vi "Waveforms.Process.vi"(0 "Data":dbl[](array[numeric]), 1 "Waveform.Ref":T1, 2 "WaveformGraph.Ref":refnum<vi>, 3 "Reset?":bool, 5 "dt":dbl, 7 "offset from start (samples)":u64, 9 "t0 at start":timestamp, 11 "error in (no error)":errorcluster, 12 "Waveforms":T5) -> (15 "error out":errorcluster)   [LabVIEW 2015, in "Station.Execution.lvlib"]
uses:
  Station.Execution.lvlib
  <vilib>/NI Veristand/Execution/WaveformStreaming/WaveformStreamSpecification.ctl
  NationalInstruments.VeriStand.ClientAPI
  <vilib>/NI Veristand/Execution/WaveformStreaming/Registered Waveform Streams Data Event Refnum (DBL).ctl
  <vilib>/NI Veristand/Execution/WaveformStreaming/Waveform Data Watcher Event Data (DBL).ctl
  <vilib>/NI Veristand/Execution/WaveformStreaming/WaveformDataWatcherDBL.ctl
  <vilib>/NI Veristand/Execution/WaveformStreaming/WaveformStreamingAPI.ctl
  <vilib>/NI Veristand/Execution/WaveformStreaming/NI_VS Waveform Streaming Interface.lvlib
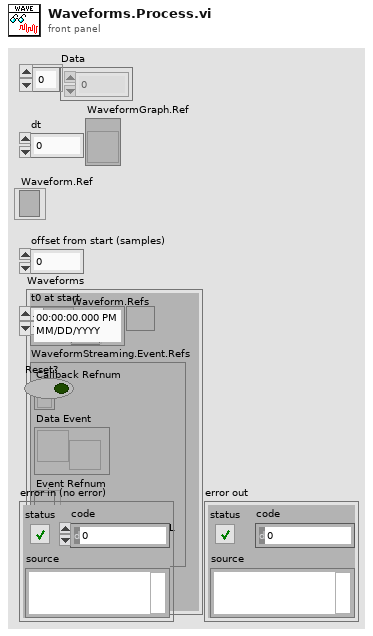
[diagram p1: front panel]
types:
  T1 = typedef "NI_VS Waveform Streaming Interface.lvlib/WaveformStreamSpecification.ctl" = refnum<k24>
  T2 = typedef "NI_VS Waveform Streaming Interface.lvlib/Registered Waveform Streams Data Event Refnum (DBL).ctl" = cluster{"Callback Refnum":refnum<k27>, "Data Event":refnum<user-event>, "Event Refnum":refnum<event-registration>, "WaveformDataWatcherDBL":T3}
  T3 = typedef "NI_VS Waveform Streaming Interface.lvlib/WaveformDataWatcherDBL.ctl" = refnum<k24>
  T4 = typedef "NI_VS Waveform Streaming Interface.lvlib/WaveformStreamingAPI.ctl" = refnum<k24>
  T5 = cluster{"Waveform.Refs":T1[], "WaveformStreaming.Event.Refs":T2, "WaveformStreaming.Ref":T4}
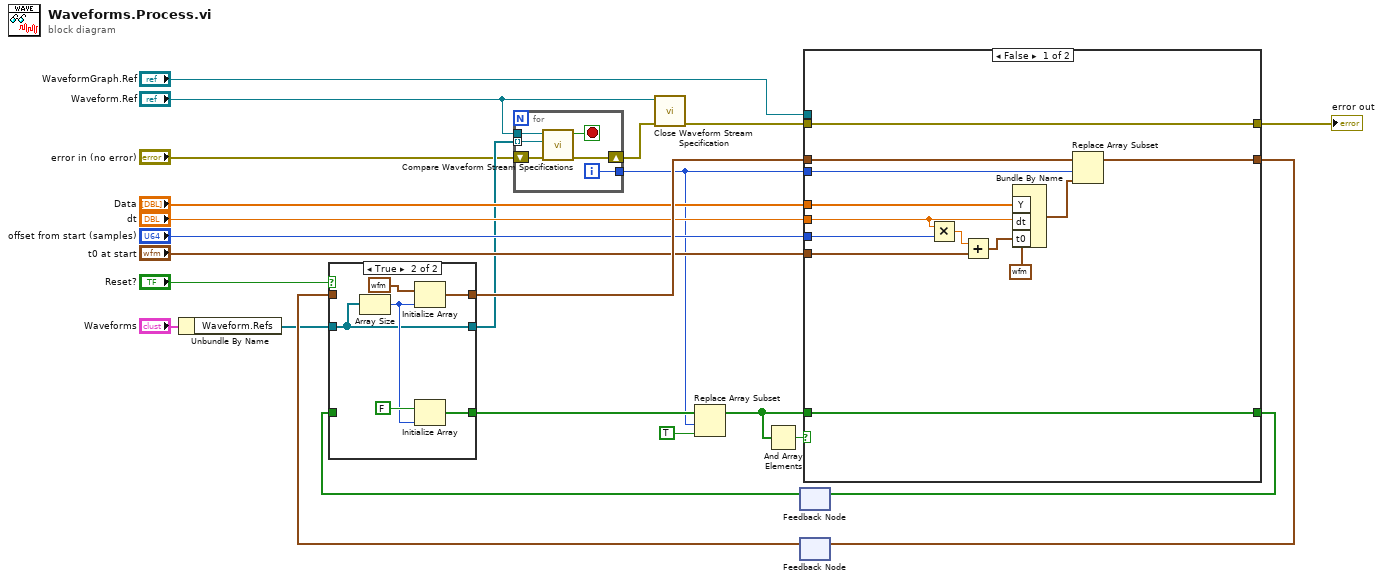
[diagram p0: block diagram]
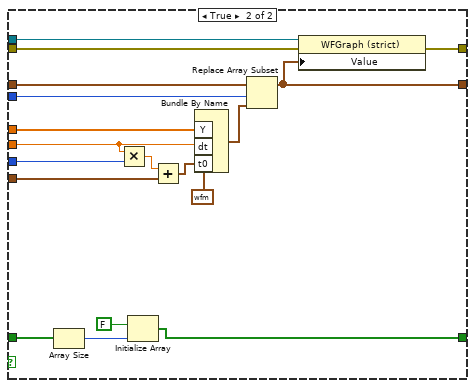
[diagram p3: hidden frame]
diagram:
  n1 = Unbundle By Name("Waveforms") -> ("Waveform.Refs"=w6:T1[])
  n2 = feedback #1() -> (w23:bool[])  [unwired: 1 in]
  n3 = feedback #2() -> (w24:waveform(dbl)[])  [unwired: 1 in]
  n4 = case shown="True" "Reset?" {
    tunnel: w6 -> [w25 w28]
    tunnel: [w27 w31] -> w19
    tunnel: [w26 w30] -> w20
    tunnel: w23 -> [w27 _]
    tunnel: w24 -> [w26 _]
    tunnel: [w25 w28] -> w5
    frame False {
    }
    frame True {
      n5 = Array Size(array=w28) -> (size(s)=w29:i32)
      n6 = Initialize Array(waveform(dbl) {"t0"=timestamp(0 s since 1904-01-01), "dt"=1.0, "Y"=[]} ("waveform"), w29) -> (w30:waveform(dbl)[])
      n7 = Initialize Array(FALSE, w29) -> (w31:bool[])
    }
  }
  n8 = for {
    tunnel: w5 -> [w39] mode=indexing
    tunnel: [w37] -> w4
    tunnel: "Waveform.Ref" -> [w36]
    shift-right: [w34] -> w1
    shift-left: "error in (no error)" -> [w35]
    i -> [w37]
    stop <- w38 stop-if-true
    n9 = call <vilib>:"Compare Waveform Stream Specifications.vi"("error in (no error)"=w35, "WaveformStreamSpecification to compare"=w39, "WaveformStreamSpecification"=w36) -> ("error out"=w34:errorcluster, "equivalent?"=w38:bool)  [unwired: 7 in]
  }
  n10 = call <vilib>:"Close Waveform Stream Specification.vi"("error in (no error)"=w1, "WaveformStreamSpecification"="Waveform.Ref") -> ("error out"=w10:errorcluster)  [unwired: 9 in]
  n11 = Replace Array Subset(array=w19, new element=TRUE ("new element/subarray"), index=w4) -> (w13:bool[])
  n12 = And Array Elements(Boolean array=w13) -> (logical AND=w12:bool)
  n13 = case shown="False" w12 {
    tunnel: w13 -> [w52 w63]
    tunnel: [w52 w60] -> w22
    tunnel: w4 -> [w51 w68]
    tunnel: w20 -> [w50 w70]
    tunnel: [w49 w69] -> w21
    tunnel: "Data" -> [w48 w67]
    tunnel: "dt" -> [w47 w66]
    tunnel: "t0 at start" -> [w46 w64]
    tunnel: "offset from start (samples)" -> [w45 w65]
    tunnel: w10 -> [w44 w59]
    tunnel: [w44 w58] -> w9
    tunnel: "WaveformGraph.Ref" -> [_ w57]
    frame False {
      n14 = Multiply(x=w47, y=w45) -> (x*y=w42:dbl)
      n15 = Add(x=w42, y=w46) -> (x+y=w43:timestamp)
      n16 = Bundle By Name(cluster=waveform(dbl) {"t0"=timestamp(0 s since 1904-01-01), "dt"=1.0, "Y"=[]} ("waveform"), "Y"=w48, "dt"=w47, "t0"=w43) -> (w40:waveform(dbl))
      n17 = Replace Array Subset(array=w50, new element=w40, index=w51) -> (w49:waveform(dbl)[])
    }
    frame True {
      n18 = Array Size(array=w63) -> (size(s)=w61:i32)
      n19 = Multiply(x=w66, y=w65) -> (x*y=w55:dbl)
      n20 = Initialize Array(FALSE, w61) -> (w60:bool[])
      n21 = Add(x=w55, y=w64) -> (x+y=w56:timestamp)
      n22 = Bundle By Name(cluster=waveform(dbl) {"t0"=timestamp(0 s since 1904-01-01), "dt"=1.0, "Y"=[]} ("waveform"), "Y"=w67, "dt"=w66, "t0"=w56) -> (w53:waveform(dbl))
      n23 = Replace Array Subset(array=w70, new element=w53, index=w68) -> (w69:waveform(dbl)[])
      n24 = property class="WFGraph (strict)"(reference=w57, error in=w59, "Value"=w69) -> (error out=w58:errorcluster)  [unwired: 1 out]
    }
  }
  "error out" <- w9
  n25 = feedback-in #1(w22) -> ()
  n26 = feedback-in #2(w21) -> ()
